vi "Pre Launch Init.vi"(11 "Measure Object in":refnum<class "Worker Actor.lvclass">) -> (0 "error out":errorcluster, 3 "Measure Object out":refnum<class "Worker Actor.lvclass">)   [LabVIEW 2021, in "Worker Actor.lvclass"]
doc: "(<B>Filename</B>: Actor Framework.lvlib:Actor.lvclass:Pre Launch Init.vi)\n\nDefines behavior that occurs after the Launch Nested Actor method is invoked but before the actor's Actor Core method begins running.\n\nBy default, this method does nothing. A descendant class may override it to define behavior."
uses:
  Worker Actor.lvclass
  Template Module/Template Module.lvclass
  Worker Actor.lvclass/Worker Actor.ctl
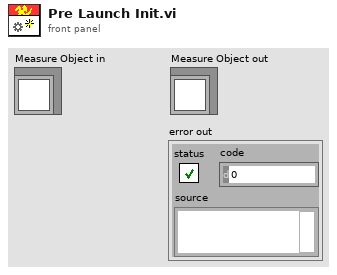
[diagram p1: front panel]
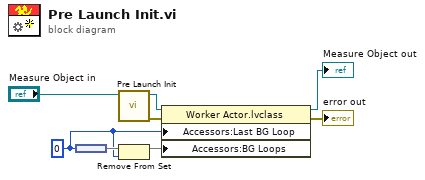
[diagram p0: block diagram]
diagram:
  w2 = 0 ("Last BG Loop")
  n1 = node(w2) -> (w3:set{i32})
  n2 = call-parent "Pre Launch Init.vi"("Measure Object in"="Measure Object in") -> ("error out"=w8:errorcluster, "Measure Object out"=w5:refnum<class "Worker Actor.lvclass">)  [unwired: 9 in]
  n3 = Remove From Set(10:w2, 11:w3) -> (3:w1:set{i32})  [unwired: 1 out]
  n4 = property class="Worker Actor.lvclass"(reference=w5, error in=w8, "Accessors:Last BG Loop"=w2, "Accessors:BG Loops"=w1) -> (reference out=→"Measure Object out":refnum<class "Worker Actor.lvclass">, error out=→"error out":errorcluster)
